vi "Get Data Name from TD.vi"(8 "error in (no error)":errorcluster, 11 "TypeDescriptor":refnum<class "TypeDescriptor.lvclass">) -> (0 "error":errorcluster, 2 "name":string, 3 "TypeDescriptor out":refnum<class "TypeDescriptor.lvclass">)   [LabVIEW 2020, in "lvdata.lvlib" / "type_descriptor.lvlib" / "TypeDescriptor.lvclass"]
doc: "Returns the name of the data described by the type string input."
uses:
  Type Descriptor/TypeDescriptor.lvclass
  C:/projects/OpenG-Variant-Data-Library/source/library/Bytes/Bytes.lvclass
  Type Descriptor/TypeDescriptor.lvclass/TypeDescriptor.ctl
  Bytes/Bytes.lvclass/Bytes.ctl
  0e45dee4-0aff-46c0-879f-09e0c5daf274.vi
  60867f29-c6a0-45b9-95f9-cabf556cf7ee.vi
  Bytes/read.vi
  Bytes/to_data.vi
  Type Descriptor/get_num_elements.vi/b3898c1b-5169-4cb1-894b-457c92b4a1c3.vi
  0e45dee4-0aff-46c0-879f-09e0c5daf274.vi/81433c74-ee36-47cf-a886-10c868675b30.vi
  0e45dee4-0aff-46c0-879f-09e0c5daf274.vi/d8d9ff34-2c15-4edb-a5ad-7260f11560db.vi
  60867f29-c6a0-45b9-95f9-cabf556cf7ee.vi/81433c74-ee36-47cf-a886-10c868675b30.vi
  60867f29-c6a0-45b9-95f9-cabf556cf7ee.vi/d8d9ff34-2c15-4edb-a5ad-7260f11560db.vi
  Bytes/from_byte_array.vi
  Type Descriptor/get_num_elements.vi/b3898c1b-5169-4cb1-894b-457c92b4a1c3.vi/81433c74-ee36-47cf-a886-10c868675b30.vi
  Type Descriptor/get_num_elements.vi/b3898c1b-5169-4cb1-894b-457c92b4a1c3.vi/d8d9ff34-2c15-4edb-a5ad-7260f11560db.vi
  Bytes/Bytes.lvclass
  <userlib>/_OpenG.lib/error/error.llb/openg_error.lvlib
  openg_variant.lvlib
  lvdata.lvlib
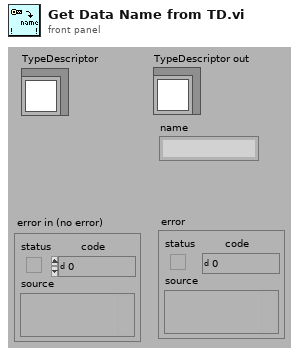
[diagram p1: front panel]
types:
  T1 = typedef "openg_variant.lvlib/Type Descriptor Enumeration.ctl" = enum8{"<Null>", "I8", "I16", "I32", "I64", "U8", "U16", "U32", "U64", "SGL", "DBL", "EXT", "CSG", "CDB", "CXT", "0x0F", "0x10", "0x11", "0x12", "0x13", "0x14", "Enum U8", "Enum U16", "Enum U32", "Enum U64", "SGL PQ", "DBL PQ", "EXT PQ", "CSG PQ", "CDB PQ", "CXT PQ", "0x1F", "0x20", "Boolean", "0x22", "0x23", "0x24", "0x25", "0x26", "0x27", "0x28", "0x29", "0x2A", "0x2B", "0x2C", "0x2D", "0x2E", "0x2F", "String", "0x31", "Path", "Pict", "0x34", "0x35", "0x36", "DAQ", "0x38", "0x39", "0x3A", "0x3B", "0x3C", "0x3D", "0x3E", "0x3F", "Array", "0x41", "0x42", "0x43", "0x44", "0x45", "0x46", "0x47", "0x48", "0x49", "0x4A", "0x4B", "0x4C", "0x4D", "0x4E", "0x4F", "Cluster", "0x51", "0x52", "Variant", "Waveform", "0x55", "0x56", "0x57", "0x58", "0x59", "0x5A", "0x5B", "0x5C", "0x5D", "0x5E", "Fixed Point", "0x60", "0x61", "0x62", "0x63", "0x64", "0x65", "0x66", "0x67", "0x68", "0x69", "0x6A", "0x6B", "0x6C", "0x6D", "0x6E", "0x6F", "Refnum", "0x71", "0x72", "Set Collection", "Map Collection"}
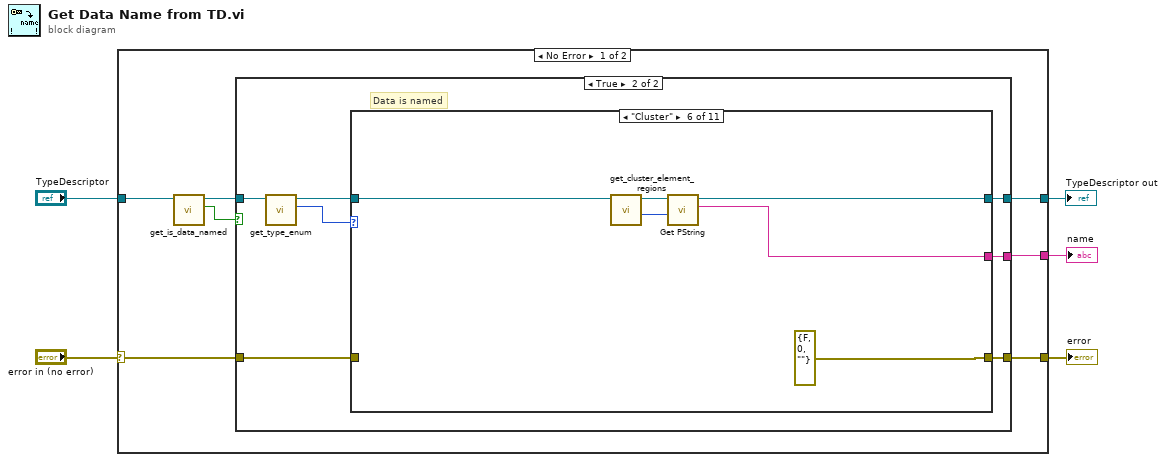
[diagram p0: block diagram]
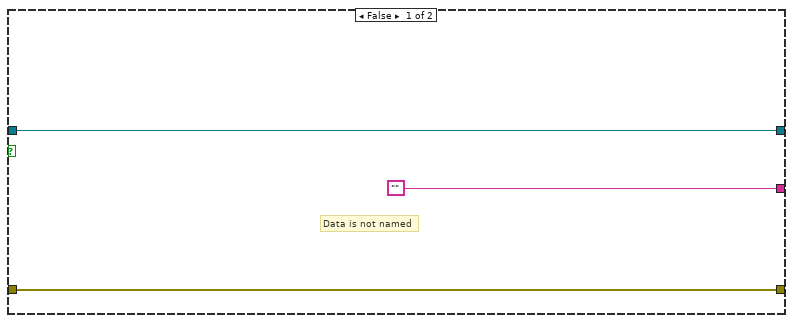
[diagram p2: hidden frame]
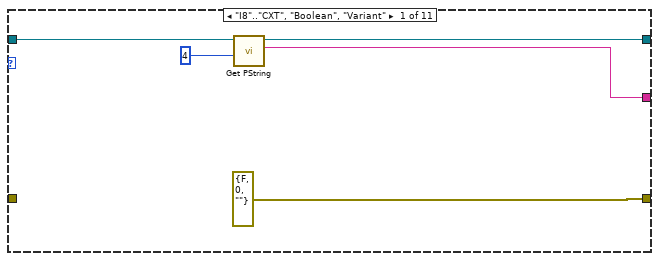
[diagram p3: hidden frame]
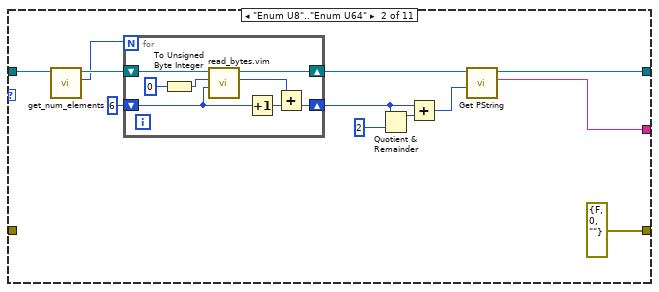
[diagram p4: hidden frame]
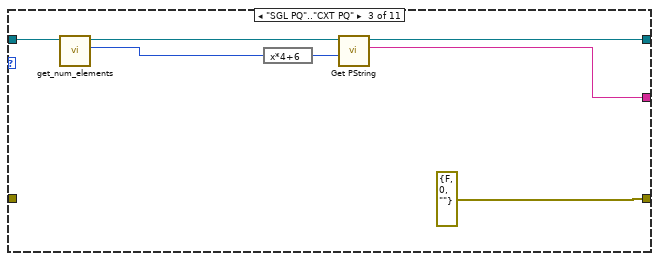
[diagram p5: hidden frame]
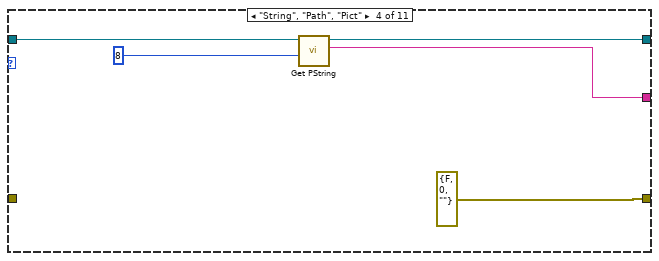
[diagram p6: hidden frame]
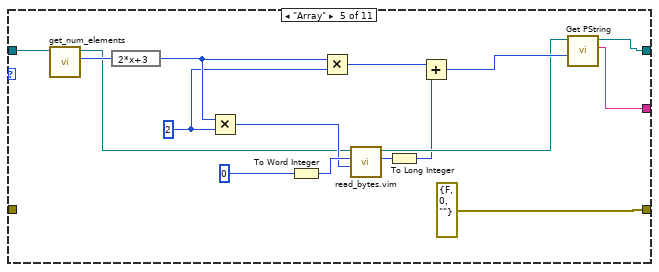
[diagram p7: hidden frame]
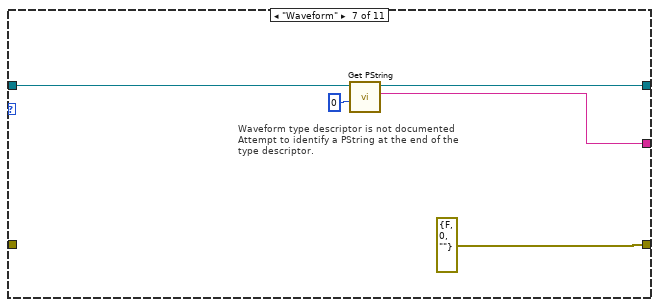
[diagram p8: hidden frame]
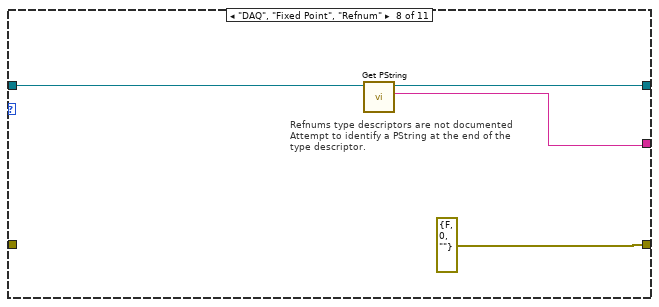
[diagram p9: hidden frame]
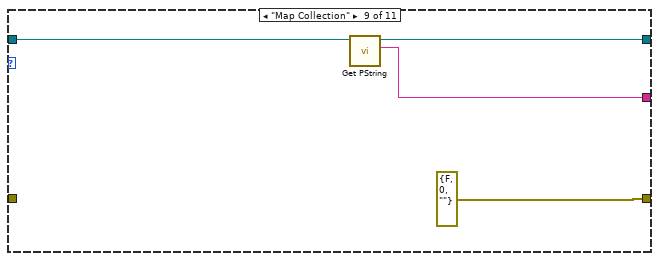
[diagram p10: hidden frame]
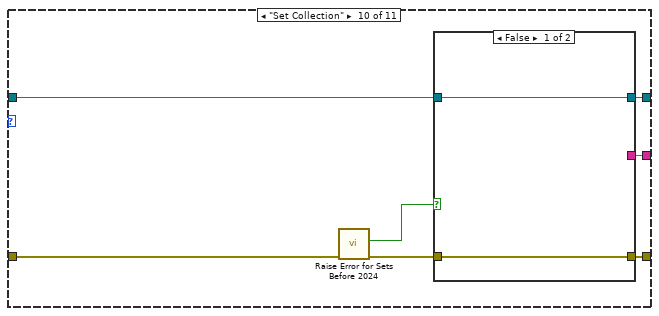
[diagram p11: hidden frame]
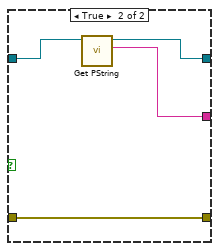
[diagram p12: hidden frame]
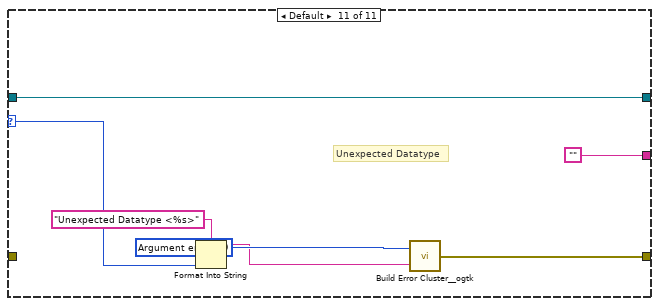
[diagram p13: hidden frame]
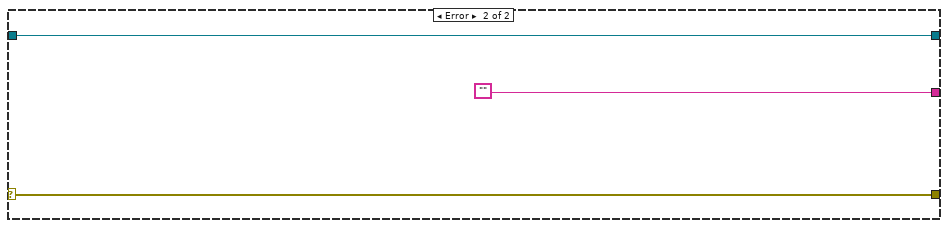
[diagram p14: hidden frame]
diagram:
  n1 = case shown="No Error" "error in (no error)" {
    selector: "error in (no error)" -> [w10 w117]
    tunnel: "TypeDescriptor" -> [w8 w116]
    tunnel: [w12 ""] -> w4
    tunnel: [w11 w117] -> w3
    tunnel: [w6 w116] -> w1
    frame No Error {
      n2 = call "get_is_data_named.vi"("TypeDescriptor in"=w8) -> ("is_named?"=w7:bool, "TypeDescriptor out"=w9:refnum<class "TypeDescriptor.lvclass">)  [unwired: 9 in]
      n3 = case shown="True" w7 {
        tunnel: [w13 w22] -> w11
        tunnel: ["" w21] -> w12
        tunnel: w9 -> [w14 w18]
        tunnel: w10 -> [w13 w20]
        tunnel: [w14 w16] -> w6
        frame False {
          # "Data is not named"
        }
        frame True {
          # "Data is named"
          n4 = call "get_type_enum.vi"("TypeDescriptor"=w18) -> ("type"=w17:T1, "TypeDescriptor out"=w19:refnum<class "TypeDescriptor.lvclass">)  [unwired: 9 in]
          n5 = case shown="\"Cluster\"" w17 {
            selector: w17 -> [_ _ _ _ _ _ _ _ _ _ w109]
            tunnel: [errorcluster {"status"=FALSE, "code"=0, "source"=""} ("error out") errorcluster {"status"=FALSE, "code"=0, "source"=""} ("error out") errorcluster {"status"=FALSE, "code"=0, "source"=""} ("error out") errorcluster {"status"=FALSE, "code"=0, "source"=""} ("error out") errorcluster {"status"=FALSE, "code"=0, "source"=""} ("error out") errorcluster {"status"=FALSE, "code"=0, "source"=""} ("error out") errorcluster {"status"=FALSE, "code"=0, "source"=""} ("error out") errorcluster {"status"=FALSE, "code"=0, "source"=""} ("error out") errorcluster {"status"=FALSE, "code"=0, "source"=""} ("error out") w100 w114] -> w22
            tunnel: [w25 w32 w53 w59 w74 w80 w85 w90 w94 w101 ""] -> w21
            tunnel: w19 -> [w24 w30 w51 w56 w62 w77 w84 w88 w92 w96 w108]
            tunnel: w20 -> [_ _ _ _ _ _ _ _ _ w98 _]
            tunnel: [w23 w28 w48 w55 w60 w76 w82 w87 w91 w95 w108] -> w16
            frame "I8".."CXT", "Boolean", "Variant" {
              n6 = call "Get PString.vi"("offset (0)"=4, "bytes"=w24) -> ("PString"=w25:string, "Bytes out"=w23:refnum<class "TypeDescriptor.lvclass">)  [unwired: 7 in, 1 out]
            }
            frame "Enum U8".."Enum U64" {
              n7 = call "get_num_elements.vi"("TypeDescriptor"=w30) -> ("num_element"=w29:i32, "TypeDescriptor out"=w31:refnum<class "TypeDescriptor.lvclass">)  [unwired: 9 in]
              n8 = for {
                N: w29 -> [_]
                shift-right: [w41] -> w38
                shift-left: 6 -> [w42]
                shift-right: [w44] -> w34
                shift-left: w31 -> [w47]
                n9 = To Unsigned Byte Integer(number=0) -> (unsigned 8bit integer=w45:u8)
                n10 = call "read_bytes.vim"("byte offset"=w42, "data type"=w45, "Bytes in"=w47) -> ("value"=w43:u8, "Bytes out"=w44:refnum<class "TypeDescriptor.lvclass">)  [unwired: 7 in]
                n11 = Increment(x=w42) -> (x+1=w40:i32)
                n12 = Add(x=w43, y=w40) -> (x+y=w41:i32)
              }
              n13 = Quotient & Remainder(x=w38, y=2) -> (x-y*floor(x/y)=w35:i32)  [unwired: 1 out]
              n14 = Add(x=w38, y=w35) -> (x+y=w33:i32)
              n15 = call "Get PString.vi"("offset (0)"=w33, "bytes"=w34) -> ("PString"=w32:string, "Bytes out"=w28:refnum<class "TypeDescriptor.lvclass">)  [unwired: 7 in, 1 out]
            }
            frame "SGL PQ".."CXT PQ" {
              n16 = call "get_num_elements.vi"("TypeDescriptor"=w51) -> ("num_element"=w49:i32, "TypeDescriptor out"=w50:refnum<class "TypeDescriptor.lvclass">)  [unwired: 9 in]
              n17 = expression code="x*4+6"(w49) -> (w54:i32)
              n18 = call "Get PString.vi"("offset (0)"=w54, "bytes"=w50) -> ("PString"=w53:string, "Bytes out"=w48:refnum<class "TypeDescriptor.lvclass">)  [unwired: 7 in, 1 out]
            }
            frame "String", "Path", "Pict" {
              n19 = call "Get PString.vi"("offset (0)"=8, "bytes"=w56) -> ("PString"=w59:string, "Bytes out"=w55:refnum<class "TypeDescriptor.lvclass">)  [unwired: 7 in, 1 out]
            }
            frame "Array" {
              w70 = u16 2 ("y")
              n20 = call "get_num_elements.vi"("TypeDescriptor"=w62) -> ("num_element"=w64:i32, "TypeDescriptor out"=w63:refnum<class "TypeDescriptor.lvclass">)  [unwired: 9 in]
              n21 = expression code="2*x+3"(w64) -> (w71:i32)
              n22 = Multiply(x=w71, y=w70) -> (x*y=w66:i32)
              n23 = To Word Integer(number=i16 0 ("y")) -> (16bit integer=w68:i16)
              n24 = Multiply(x=w71, y=w70) -> (x*y=w73:i32)
              n25 = call "read_bytes.vim"("byte offset"=w66, "data type"=w68, "Bytes in"=w63) -> ("value"=w65:i16, "Bytes out"=w67:refnum<class "TypeDescriptor.lvclass">)  [unwired: 7 in]
              n26 = To Long Integer(number=w65) -> (32bit integer=w61:i32)
              n27 = Add(x=w73, y=w61) -> (x+y=w72:i32)
              n28 = call "Get PString.vi"("offset (0)"=w72, "bytes"=w67) -> ("PString"=w74:string, "Bytes out"=w60:refnum<class "TypeDescriptor.lvclass">)  [unwired: 7 in, 1 out]
            }
            frame "Cluster" {
              n29 = call "get_cluster_element_regions.vi"("TypeDescriptor"=w77) -> ("offset past element TDs"=w79:i32, "TypeDescriptor out"=w78:refnum<class "TypeDescriptor.lvclass">)  [unwired: 8 in, 1 out]
              n30 = call "Get PString.vi"("offset (0)"=w79, "bytes"=w78) -> ("PString"=w80:string, "Bytes out"=w76:refnum<class "TypeDescriptor.lvclass">)  [unwired: 7 in, 1 out]
            }
            frame "Waveform" {
              # "Waveform type descriptor is not documented\nAttempt to identify a PString at the end of the\ntype descriptor."
              n31 = call "Get PString.vi"("offset (0)"=0, "bytes"=w84) -> ("PString"=w85:string, "Bytes out"=w82:refnum<class "TypeDescriptor.lvclass">)  [unwired: 7 in, 1 out]
            }
            frame "DAQ", "Fixed Point", "Refnum" {
              # "Refnums type descriptors are not documented\nAttempt to identify a PString at the end of the\ntype descriptor."
              n32 = call "Get PString.vi"("bytes"=w88) -> ("PString"=w90:string, "Bytes out"=w87:refnum<class "TypeDescriptor.lvclass">)  [unwired: 8 in, 1 out]
            }
            frame "Map Collection" {
              n33 = call "Get PString.vi"("bytes"=w92) -> ("PString"=w94:string, "Bytes out"=w91:refnum<class "TypeDescriptor.lvclass">)  [unwired: 8 in, 1 out]
            }
            frame "Set Collection" {
              n34 = call "Raise Error for Sets Before 2024.vi"("error in (no error)"=w98) -> ("error out"=w97:errorcluster, "supported?"=w99:bool)  [unwired: 9 in]
              n35 = case shown="False" w99 {
                tunnel: w96 -> [w102 w105]
                tunnel: [_ w107] -> w101
                tunnel: [w103 w106] -> w100
                tunnel: w97 -> [w103 w106]
                tunnel: [w102 w104] -> w95
                frame False {
                }
                frame True {
                  n36 = call "Get PString.vi"("bytes"=w105) -> ("PString"=w107:string, "Bytes out"=w104:refnum<class "TypeDescriptor.lvclass">)  [unwired: 8 in, 1 out]
                }
              }
            }
            frame Default {
              w113 = 1 items=["No error", "Argument error", "Memory is full", "Out of zone", "End of file", "File already open", "Generic file I/O error", "File not found", "File permission error", "Disk is full", "Duplicate path", "Too many files open", "System feature not enabled", "Resource file not found", "Cannot add resource", "Resource not found", "Image not found", "Image memory error", "Pen does not exist", "Config type invalid", "Config token not found", "Config parse error", "Config memory error", "Bad external code format", "Bad external code offset", "External code not present", "Null window", "Destroy window error", "Null menu", "Print aborted", "Bad print record", "Print driver error", "Windows error during printing", "Memory error during printing", "Print dialog error", "Generic print error", "Invalid device refnum", "Device not found", "Device parameter error", "Device unit error", "Cannot open device", "Device call aborted", "Generic error", "Cancelled by user", "Object ID too low", "Object ID too high", "Object not in heap", "Unknown heap", "Unknown object (invalid DefProc)", "Unknown object (DefProc not in table)", "Message out of range", "Invalid (null) method", "Unknown message", "Manager call not supported", "Bad address", "Network operation in progress", "Network operation timed out", "Connection is busy", "Network attribute not supported", "Network error", "Address in use", "System out of memory", "Connection aborted", "Connection refused", "Not connected", "Already connected", "Connection closed", "Initialization error (interapplication manager)", "Bad occurrence", "Wait on unbound occurrence handler", "Occurrence queue overflow", "Datalog type conflict", "Unused", "Unrecognized type (interapplication manager)", "Memory corrupt", "Failed to make temporary DLL", "Old CIN version", "Drag socket not found", "Failed to load drop-object", "Failed to register OLE object", "Failed to release OLE object", "Format specifier type mismatch", "Unknown format specifier", "Too few format specifiers", "Too many format specifiers", "Scan failed", "Newer CIN version", "Error converting to variant", "Runtime menu error", "Password tampered", "Variant attribute not found", "Incompatible variant data type", "Event data is not available", "Event Store is not present", "Occurrence is not found", "Event Queue is not created", "Event info is not available", "Refnum passed is NULL", "Error retrieving Class GUID", "Error retrieving CoClass GUID", "Error retrieving TypeLib GUID.", "Bad built application magic bytes.", "Specific driver is different from the specific driver associated with the Logical Name.", "There is no session opened to the class driver.", "Max Error", "MAX - Error with config objects", "MAX - Error loading configuration", "MAX - Group not supported"]
              # "Unexpected Datatype"
              n37 = Format Into String(format string="Unexpected Datatype <%s>" ("Format String"), w109) -> (resulting string=w110:string)  [unwired: 2 in, 1 out]
              n38 = call <userlib>:"Build Error Cluster__ogtk.vi"("String to Prepend to source (\"\")"=w110, "code"=w113) -> ("error out"=w114:errorcluster)
            }
          }
        }
      }
    }
    frame Error {
    }
  }
  "name" <- w4
  "error" <- w3
  "TypeDescriptor out" <- w1
